vi "Sort Paths.vi"(0 "unsorted array":string[](array[string]), 11 "error in":errorcluster) -> (4 "Table data":string[][](array[string]), 6 "sorted array":string[](array[string]), 15 "error out":errorcluster)   [LabVIEW 2020, in "Custom Sort Function.lvlib"]
doc: "This VI gets in string array as input and sorts it as per our requirement"
uses:
  Libraries/Custom Sort Function.lvlib
  e74950d2-8bb2-46d1-9d88-96c127758961.vi
  <vilib>/Comparison/Less/Less Functor/Less Functor.lvclass
panel:
  # "SORT ARRAY WITH SERIAL NUMBER"
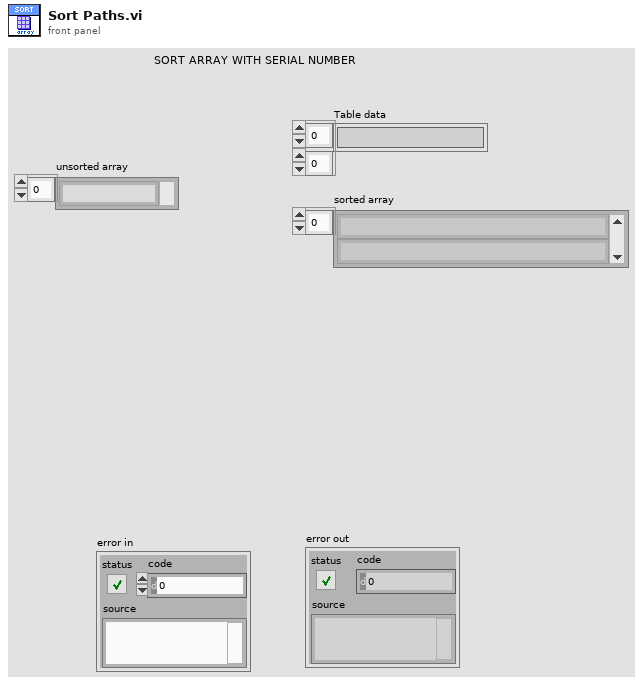
[diagram p1: front panel]
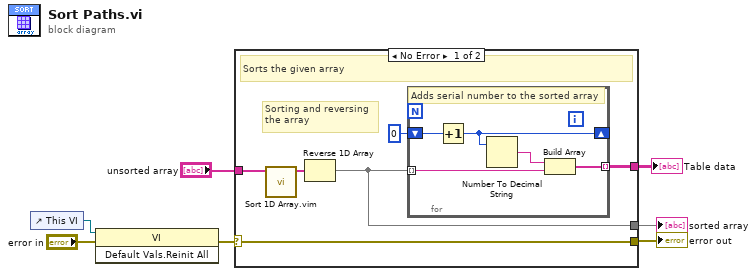
[diagram p0: block diagram]
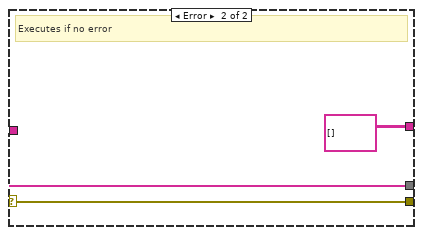
[diagram p2: hidden frame]
diagram:
  n1 = control-ref of="This VI"() -> (w3:refnum<vi>)
  n2 = invoke class="VI" method="Default Vals.Reinit All"(reference=w3, error in="error in") -> (error out=w2:errorcluster)  [unwired: 1 in, 2 out]
  n3 = case shown="No Error" w2 {
    selector: w2 -> [w12 w19]
    tunnel: [w12 w19] -> w7
    tunnel: [w10 string[][] []] -> w6
    tunnel: "unsorted array" -> [w9 w21]
    tunnel: [w8 w21] -> w4
    frame No Error {
      # "Sorting and reversing\nthe array"
      # "Sorts the given array"
      n4 = call "Sort 1D Array.vim"("unsorted array"=w9) -> ("sorted array"=w13:string[])  [unwired: 10 in]
      n5 = Reverse 1D Array(array=w13) -> (reversed array=w8:string[])
      n6 = for {
        tunnel: w8 -> [w15] mode=indexing
        shift-right: [w17] -> _
        shift-left: 0 -> [w18]
        tunnel: [w14] -> w10 mode=indexing
        # "Adds serial number to the sorted array"
        n7 = Increment(x=w18) -> (x+1=w17:i32)
        n8 = Number To Decimal String(number=w17) -> (decimal integer string=w16:string)  [unwired: 1 in]
        n9 = Build Array(w16, w15) -> (w14:string[])
      }
    }
    frame Error {
      # "Executes if no error"
    }
  }
  "error out" <- w7
  "sorted array" <- w4
  "Table data" <- w6
